vi "Structure.vi"(8 "error in":errorcluster, 11 "reference":refnum<vi>) -> (0 "error out":errorcluster, 3 "structure out":refnum<class "Structure.lvclass">)   [LabVIEW 2014, in "Structure.lvclass"]
uses:
  Structure.lvclass
  CaseStructure/CaseStructure.lvclass
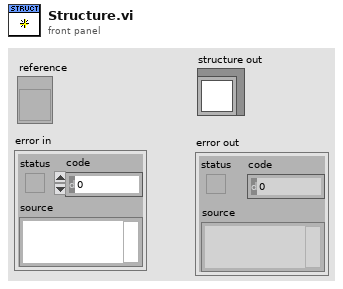
[diagram p1: front panel]
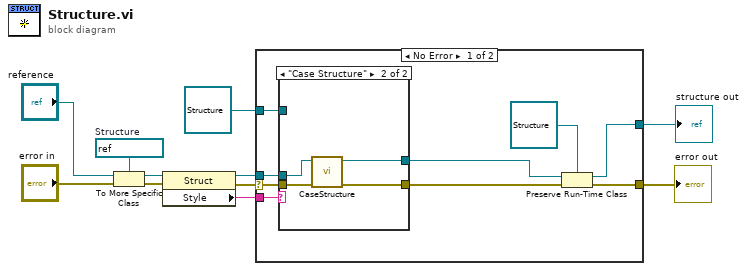
[diagram p0: block diagram]
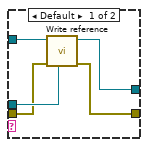
[diagram p2: hidden frame]
diagram:
  w11 = refnum<vi> refnum  # Structure
  n1 = To More Specific Class(target class=w11, reference="reference", error in="error in") -> (specific class reference=w10:refnum<vi>, error out=w9:errorcluster)
  n2 = property class="Struct"(reference=w10, error in=w9) -> (reference out=w7:refnum<vi>, error out=w2:errorcluster, "Style"=w8:string)
  n3 = case shown="No Error" w2 {
    selector: w2 -> [w15 w30]
    tunnel: w8 -> [w20 _]
    tunnel: w7 -> [w19 _]
    tunnel: [w17 _] -> w4
    tunnel: [w16 w30] -> w3
    tunnel: refnum<class "Structure.lvclass"> refnum ("structure out") -> [w14 _]
    frame No Error {
      n4 = case shown="\"Case Structure\"" w20 {
        tunnel: [w24 w27] -> w13
        tunnel: w19 -> [w23 w28]
        tunnel: w15 -> [w22 w29]
        tunnel: [w21 w26] -> w12
        tunnel: w14 -> [w25 _]
        frame Default {
          n5 = call-dynamic "Write reference.vi"("reference"=w23, "error in"=w22, "GObject in"=w25) -> ("error out"=w21:errorcluster, "GObject out"=w24:refnum<class "Structure.lvclass">)  [unwired: 5 in]
        }
        frame "Case Structure" {
          n6 = call "CaseStructure.vi"("error in"=w29, "reference"=w28) -> ("error out"=w26:errorcluster, "CaseStructure out"=w27:refnum<class "CaseStructure.lvclass">)  [unwired: 8 in]
        }
      }
      n7 = Preserve Run-Time Class(object in=w13, error in=w12, 2:refnum<class "Structure.lvclass"> refnum ("structure out")) -> (object out=w17:refnum<class "Structure.lvclass">, error out=w16:errorcluster)
    }
    frame Error {
    }
  }
  "error out" <- w3
  "structure out" <- w4
